vi "Eval Condition.vi"(7 "Variables":refnum<class "Variables.lvclass">, 8 "error in (no error)":errorcluster, 9 "Sequence Time":T1, 11 "OutOfRange Condition in":refnum<class "OutOfRange Condition.lvclass">) -> (0 "error out":errorcluster, 2 "Result":bool, 3 "OutOfRange Condition out":refnum<class "OutOfRange Condition.lvclass">)   [LabVIEW 2020, in "VolatusSeq.lvlib" / "OutOfRange Condition.lvclass"]
uses:
  OutOfRange Condition.lvclass
  Sequence Time.ctl
  Variables/Variables.lvclass
  OutOfRange Condition.lvclass/OutOfRange Condition.ctl
  lv-vecto/Vecto/Channel DBL/Channel DBL.lvclass/Channel DBL.ctl
  lv-vecto/Vecto/Group DBL/Value by Index.vi
  Condition Value/Condition Value.lvclass
  VolatusSeq.lvlib
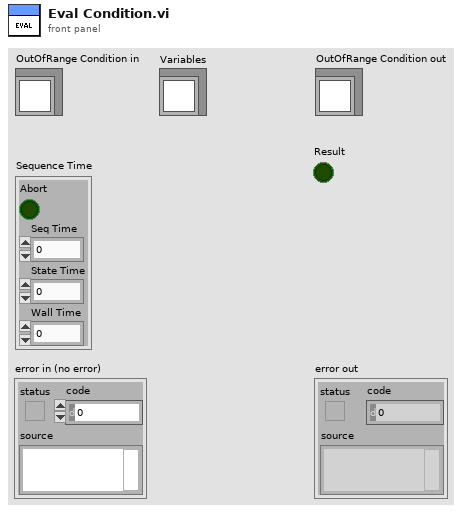
[diagram p1: front panel]
types:
  T1 = typedef "VolatusSeq.lvlib/Sequence Time.ctl" = cluster{"Abort":bool, "Seq Time":dbl, "State Time":dbl, "Wall Time":dbl}
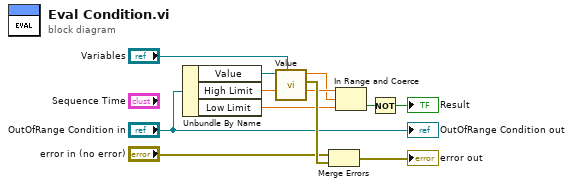
[diagram p0: block diagram]
diagram:
  n1 = Unbundle By Name("OutOfRange Condition in") -> ("Value"=w6:refnum<class "Condition Value.lvclass">, "High Limit"=w8:dbl, "Low Limit"=w7:dbl)
  n2 = call "Value.vi"("Variables"="Variables", "Condition Value in"=w6) -> ("error out"=w11:errorcluster, "Value"=w5:dbl)  [unwired: 8 in]
  n3 = Merge Errors("error in (no error)", w11) -> (→"error out":errorcluster)
  n4 = In Range and Coerce(upper limit=w8, x=w5, lower limit=w7) -> (In Range?=w4:bool)  [unwired: 1 out]
  n5 = Not(x=w4) -> (.not. x?=→"Result":bool)
  "OutOfRange Condition out" <- "OutOfRange Condition in"
